vi "HFRR ADV v09.vi"() -> ()   [LabVIEW 2025] (continued)
                    n2657 = Get Date/Time In Seconds() -> (seconds since 1Jan1904=w3395:timestamp)
                    n2658 = To Double Precision Float(number=w3395) -> (double precision float=w3393:dbl)
                    n2659 = local write "acq timer"(w3393) -> ()
                    n2660 = local write "act save time"(w3393) -> ()
                  }
                }
                n2661 = call "Elapsed Time"("Time Target (s)"="Countdown", "Reset"=w3299) -> ("Elapsed Time (s)"=w3304:dbl, "Time has Elapsed"=w3302:bool)  [unwired: 10 in, 6 out]
                "Countdown 2" <- w3304
                n2662 = Subtract(x=w3304, y=2.0) -> (x-y=w3307:dbl)
                n2663 = Less?(x=w3307, y="Countdown") -> (x < y?=w3305:bool)
                n2664 = And(x=w3305, y=w3302) -> (x .and. y?=w3301:bool)
                n2665 = case shown="True" w3301 {
                  frame False {
                  }
                  frame True {
                    (unwired) dbl[] [] ("History Data")
                    n2666 = local write "Engage"(FALSE ("Engage")) -> ()
                    n2667 = local write "RUN"(TRUE ("RUN")) -> ()
                    n2668 = local read "Humidity ( %RH )"() -> (→"Rh Before":dbl)
                  }
                }
                n2669 = local read "Test \nStatus"() -> (w3297:bool)
                n2670 = Select(t=w3295, s=w3297, f=0.0) -> (s? t:f=w3296:dbl)
                n2671 = local write "Frequency ( Hz )"(w3296) -> ()
                n2672 = local write "Freq"(w3296) -> ()
              }
              frame #1 {
                w3418 = 1000000.0 ("x")
                # "Elapsed time\ncof\nstroke\nAir temp\nTemp\nHumidity"
                # "acq timer\n\nact save time"
                # "convert to microseconds"
                n2673 = local read "COUNT"() -> (w3401:i32)
                n2674 = local read "Rate"() -> (w3414:dbl)
                n2675 = Divide(x=w3418, y=w3414) -> (x/y=w3419:dbl)
                n2676 = Greater Or Equal?(x=w3401, y=250) -> (x >= y?=w3400:bool)
                n2677 = Get Date/Time In Seconds() -> (seconds since 1Jan1904=w3421:timestamp)
                n2678 = case shown="True" w3400 {
                  frame False {
                    n2679 = local read "COUNT"() -> (w3422:i32)
                    n2680 = Increment(x=w3422) -> (x+1=w3423:i32)
                    n2681 = local write "COUNT"(w3423) -> ()
                  }
                  frame True {
                    n2682 = local write "COUNT"(0 ("COUNT")) -> ()
                  }
                }
                n2683 = local read "Samplingtime 2"() -> (w3399:dbl)
                n2684 = local read "act save time"() -> (w3416:dbl)
                n2685 = Divide(x=w3419, y=w3418) -> (x/y=w3417:dbl)
                n2686 = To Double Precision Float(number=w3421) -> (double precision float=w3410:dbl)
                n2687 = Add(x=w3416, y=w3399) -> (x+y=w3415:dbl)
                n2688 = local read "acq timer"() -> (w3420:dbl)
                n2689 = local read "COUNT"() -> (w3403:i32)
                n2690 = Greater Or Equal?(x=w3410, y=w3415) -> (x >= y?=w3398:bool)
                n2691 = Multiply(x=w3417, y=w3403) -> (x*y=w3409:dbl)
                n2692 = Subtract(x=w3410, y=w3420) -> (x-y=w3412:dbl)
                n2693 = local read "Save"() -> (w3413:bool)
                n2694 = Add(x=w3412, y=w3409) -> (x+y=w3396:dbl)
                "Elapsed time 3" <- w3396
                n2695 = And(x=w3398, y=w3413) -> (x .and. y?=w3411:bool)
                n2696 = Divide(x=w3396, y=60.0) -> (x/y=w3407:dbl)
                n2697 = local read "Test \nStatus"() -> (w3397:bool)
                n2698 = local read "clk"() -> (w3404:dbl)
                n2699 = Equal?(x=w3404, y=10.0) -> (x = y?=w3406:bool)
                n2700 = case shown="True" w3411 {
                  tunnel: w3410 -> [_ w3525]
                  tunnel: [FALSE ("Boolean 2") TRUE ("Boolean 2")] -> _
                  frame False {
                  }
                  frame True {
                    w3472 = ";" ("Substring")
                    # "Pid out/\nFreq response value"
                    n2701 = local write "act save time"(w3525) -> ()
                    n2702 = local read "FILE"() -> (w3466:string)
                    n2703 = call "file check.vi"("file name in"=w3466) -> ("error out"=w3469:errorcluster, "file name out"=w3464:string)  [unwired: 9 in]
                    n2704 = call "FILE PATH CREATION.vi"("error in"=w3469, "FILE NAME :"=w3464) -> ("FILE OUT"=w3467:path)  [unwired: 8 in, 1 out]
                    n2705 = Concatenate Strings(w3464, ".dgf" ("Substring")) -> (w3468:string)
                    n2706 = local read "Set Strk"() -> (w3496:dbl)
                    n2707 = local read "Stroke"() -> (w3487:dbl)
                    n2708 = local read "FF 2"() -> (→"Frictional Force ( N )" →"Frictional Force ( N )":dbl)
                    n2709 = Build Path(base path=w3467, name or relative path=w3468) -> (appended path=w3463:path)
                    n2710 = Subtract(x=w3487, y=w3496) -> (x-y=w3493:dbl)
                    n2711 = local read "COF 2"() -> (w3478:dbl)
                    "cof" <- w3478
                    "Coefficient of Friction" <- w3478
                    "COF 4" <- w3478
                    "Coefficient of Friction" <- w3478
                    n2712 = Multiply(x=w3493, y=0.05) -> (x*y=w3495:dbl)
                    n2713 = local read "TEMP"() -> (w3482:dbl)
                    "Temp" <- w3482
                    "Temperature ( Deg C )" <- w3482
                    n2714 = Add(x=w3495, y=w3496) -> (x+y=w3476:dbl)
                    "Stroke Ln" <- w3476
                    "Disp" <- w3476
                    n2715 = local read "ecr"() -> (w3479:dbl)
                    "Electrical Contact Resistance ( % )" <- w3479
                    n2716 = local read "Humidity ( %RH )"() -> (w3481:dbl)
                    "Humidity ( %RH )" <- w3481
                    "Humidity ( %RH )" <- w3481
                    n2717 = local read "Frequency ( Hz )"() -> (w3489:dbl)
                    n2718 = local read "Elapsed time"() -> (w3518:dbl)
                    n2719 = disable-structure shown="Disabled" {
                      frame Disabled {
                        n2720 = local read "ecr 3"() -> ()  [unwired: 1 in]
                      }
                      frame Enabled {
                      }
                    }
                    n2721 = local read "AIR TEMP"() -> (w3486:dbl)
                    n2722 = local read "PID-out"() -> (w3492:dbl)
                    n2723 = local write "Temperature ( Deg C )"(w3482) -> ()
                    n2724 = local write "Electrical Contact Resistance ( % )"(w3479) -> ()
                    n2725 = Number To Fractional String(number=w3476, width (-)=i16 9 ("precision (6)"), precision (6)=i16 6) -> (F-format string=w3511:string)  [unwired: 1 in]
                    n2726 = Number To Fractional String(number=w3486, width (-)=i16 9 ("precision (6)"), precision (6)=i16 3) -> (F-format string=w3510:string)  [unwired: 1 in]
                    n2727 = Number To Fractional String(number=w3482, width (-)=i16 9 ("precision (6)"), precision (6)=i16 3) -> (F-format string=w3507:string)  [unwired: 1 in]
                    n2728 = Number To Fractional String(number=w3481, width (-)=i16 9 ("precision (6)"), precision (6)=i16 3) -> (F-format string=w3504:string)  [unwired: 1 in]
                    n2729 = Number To Fractional String(number=w3479, width (-)=i16 9 ("precision (6)"), precision (6)=i16 3) -> (F-format string=w3501:string)  [unwired: 1 in]
                    n2730 = Number To Fractional String(number=w3492, width (-)=i16 9 ("precision (6)"), precision (6)=i16 3) -> (F-format string=w3497:string)  [unwired: 1 in]
                    n2731 = Number To Fractional String(number=w3489, width (-)=i16 9 ("precision (6)"), precision (6)=i16 3) -> (F-format string=w3488:string)  [unwired: 1 in]
                    n2732 = Number To Fractional String(number=w3478, width (-)=i16 9 ("precision (6)"), precision (6)=i16 6) -> (F-format string=w3519:string)  [unwired: 1 in]
                    n2733 = Number To Fractional String(number=w3518, width (-)=i16 14 ("precision (6)"), precision (6)=i16 3) -> (F-format string=w3520:string)  [unwired: 1 in]
                    n2734 = Bundle("y"=1.02, w3476, "y"=0.98) -> (w3480:cluster{"y":dbl, dbl, "y":dbl})  [unwired: 1 in]
                    n2735 = Number To Fractional String(number="Ambient Humidity :", width (-)=i16 9 ("precision (6)"), precision (6)=i16 6) -> (F-format string=w3470:string)  [unwired: 1 in]
                    n2736 = local read "RUN"() -> (w3477:bool)
                    n2737 = case shown="True" w3477 {
                      tunnel: w3480 -> [_ w3530]
                      tunnel: w3476 -> [_ w3529]
                      tunnel: w3476 -> [_ w3528]
                      tunnel: w3476 -> [_ w3527]
                      frame False {
                      }
                      frame True {
                        "Stroke ( mm )" <- w3530
                        "Stroke ( mm )" <- w3530
                        "Stroke 4" <- w3529
                        "Stroke 3" <- w3528
                        "Stroke 2" <- w3527
                      }
                    }
                    n2738 = Concatenate Strings(w3520, w3472, w3519, w3472, w3511, w3472, w3510, w3472, w3507, w3472, w3504, w3472, w3501, w3472, w3497, w3472, w3488, w3472, w3470, "\r") -> (w3517:string)
                    n2739 = call <vilib>:"Write Characters To File.vi"("append to file? (new file:F)"=TRUE, "character string"=w3517, "file path (dialog if empty)"=w3463) -> ()  [unwired: 2 in, 1 out]
                    "refresh flag" <- TRUE ("refresh flag")
                  }
                }
                n2740 = case shown="True" w3397 {
                  tunnel: w3407 -> [_ w3433]
                  tunnel: w3412 -> [_ w3443]
                  tunnel: [0.0 w3439] -> _
                  tunnel: w3406 -> [_ w3438]
                  tunnel: [0.0 w3437] -> _
                  tunnel: w3396 -> [_ w3437]
                  tunnel: w3410 -> [w3426 _]
                  frame False {
                    n2741 = local write "acq timer"(w3426) -> ()
                    n2742 = local write "Test Duration Status"(0.0 ("Test Duration Status")) -> ()
                  }
                  frame True {
                    n2743 = local read "Set Hz"() -> (w3440:dbl)
                    n2744 = local write "Elapsed time"(w3433) -> ()
                    n2745 = local read "test time"() -> (w3432:dbl)
                    n2746 = Multiply(x=w3443, y=w3440) -> (x*y=w3442:dbl)
                    n2747 = case shown="False" w3438 {
                      tunnel: w3442 -> [w3444 _]
                      tunnel: [w3444 1.0] -> w3439
                      frame False {
                        n2748 = local write "Cycles elapsed"(w3444) -> ()
                      }
                      frame True {
                      }
                    }
                    n2749 = Greater?(x=w3433, y=w3432) -> (0:w3441:bool)
                    n2750 = Subtract(x=w3432, y=w3433) -> (x-y=w3431:dbl)
                    "time" <- w3431
                    n2751 = Multiply(x=w3431, y=60.0) -> (x*y=w3430:dbl)
                    n2752 = local write "Time Remaining"(w3430) -> ()
                    n2753 = local write "Remaining Time"(w3430) -> ()
                    n2754 = case shown="True" w3441 {
                      frame False {
                      }
                      frame True {
                        w3446 = T15."Enabled" ("Disabled")
                        w3450 = "" ("FILE")
                        w3451 = TRUE ("Visible")
                        n2755 = local write "Humidity"(FALSE ("Humidity")) -> ()
                        n2756 = local write "RUN"(FALSE ("OK Button 2")) -> ()
                        n2757 = local write "Heater Button"(FALSE ("Heater Button")) -> ()
                        n2758 = local write "Auto Start Test"(FALSE ("Auto Start Test")) -> ()
                        n2759 = local write "TestCompFlg"(TRUE ("StpFlg")) -> ()
                        n2760 = local read "Humidity ( %RH )"() -> (→"Rh After":dbl)
                        n2761 = property on="STOP 2" class="Bool (strict)"("Disabled"=u8 0) -> ()  [unwired: 2 in, 2 out]
                        n2762 = local read "EVENT LOG"() -> (w3456:string)
                        n2763 = call "Event Log.vi"("Content"="Test Completed", "EVENT LOG"=w3456) -> ("EVENT LOG"=w3455:string)  [unwired: 8 in, 1 out]
                        n2764 = property on="RUN" class="Bool (strict)"("Visible"=w3451) -> ()  [unwired: 2 in, 2 out]
                        n2765 = property on="Auto Start Test" class="Bool (strict)"("Visible"=w3451) -> ()  [unwired: 2 in, 2 out]
                        n2766 = local write "Batch Ref Num :"(w3450) -> ()
                        n2767 = local write "FILE"(w3450) -> ()
                        n2768 = local write "EVENT LOG"(w3455) -> ()
                        n2769 = local write "TEST FILE NAM,E SAVED"(FALSE ("TEST FILE NAM,E SAVED")) -> ()
                        n2770 = local write "Fuel Discription :"(w3450) -> ()
                        n2771 = local write "Remarks :"(w3450) -> ()
                        n2772 = local write "Main Dashboard Buttons"(T1."Imaging" ("Main Dashboard Buttons")) -> ()
                        n2773 = local write "Main Tab"(T2."Adv Scar" ("Main Tab")) -> ()
                        n2774 = property on="FRICVALZ 2" class="Bool (strict)"("DisabledEnum"=w3446) -> ()  [unwired: 2 in, 2 out]
                        n2775 = property on="FRICVALZ 3" class="Bool (strict)"("DisabledEnum"=w3446) -> ()  [unwired: 2 in, 2 out]
                        n2776 = property on="FRICVALZ 4" class="Bool (strict)"("DisabledEnum"=w3446) -> ()  [unwired: 2 in, 2 out]
                      }
                    }
                    n2777 = Divide(x=w3433, y=w3432) -> (x/y=w3436:dbl)
                    n2778 = Multiply(x=w3436, y=100.0) -> (x*y=w3434:dbl)
                    n2779 = local write "Test Duration Status"(w3434) -> ()
                  }
                }
              }
              frame #2 {
                n2780 = case shown="True" "Heater Button" {
                  tunnel: [0.0 ("output") w3554] -> w3531
                  frame False {
                    w3534 = TRUE ("tmpchk")
                    n2781 = local read "TEMP"() -> (w3535:dbl)
                    n2782 = local write "Temp ini"(w3535) -> ()
                    n2783 = local write "Reset 4"(w3534) -> ()
                    n2784 = local write "tmpchk"(w3534) -> ()
                    n2785 = local write "reinit"(TRUE ("reinit")) -> ()
                    n2786 = local write "manual temp log"(TRUE ("manual temp log")) -> ()
                  }
                  frame True {
                    # "Logic to turn off\nthe heater when \ntemp is not rising.\nTime - 60 sec\nDelta t- 5°c"
                    n2787 = local read "Temp ini"() -> (w3542:dbl)
                    n2788 = local read "Auto Start Test"() -> (w3538:bool)
                    n2789 = Less?(x=w3542, y=53.0) -> (x < y?=w3540:bool)
                    n2790 = case shown="False" w3538 {
                      frame False {
                        n2791 = local read "Set Temp"() -> (w3565:dbl)
                        n2792 = local read "TEMP"() -> (w3564:dbl)
                        n2793 = Subtract(x=w3565, y=w3564) -> (x-y=w3563:dbl)
                        n2794 = Absolute Value(x=w3563) -> (abs(x)=w3562:dbl)
                        n2795 = Less?(x=w3562, y=0.5) -> (x < y?=w3560:bool)
                        n2796 = case shown="True" w3560 {
                          tunnel: "manual temp log" -> [_ w3566]
                          frame False {
                          }
                          frame True {
                            n2797 = case shown="True" w3566 {
                              selector: w3566 -> [_ w3567]
                              frame False {
                              }
                              frame True {
                                # "#Event log"
                                n2798 = Not(x=w3567) -> (.not. x?=w3568:bool)
                                n2799 = local write "manual temp log"(w3568) -> ()
                                n2800 = local read "EVENT LOG"() -> (w3571:string)
                                n2801 = call "Event Log.vi"("Content"="Target Temperature reached", "EVENT LOG"=w3571) -> ("EVENT LOG"=w3570:string)  [unwired: 8 in, 1 out]
                                n2802 = local write "EVENT LOG"(w3570) -> ()
                              }
                            }
                          }
                        }
                      }
                      frame True {
                        n2803 = local write "manual temp log"(TRUE ("manual temp log")) -> ()
                      }
                    }
                    n2804 = And(x="tmpchk", y=w3540) -> (x .and. y?=w3543:bool)
                    n2805 = case shown="True" w3543 {
                      frame False {
                      }
                      frame True {
                        n2806 = call "Elapsed Time8"("Time Target (s)"=300.0, "Reset"="Reset 4") -> ("Time has Elapsed"=w3573:bool)  [unwired: 10 in, 7 out]
                        n2807 = flat-sequence {
                          tunnel: w3573 -> [_]
                          frame #0 {
                            n2808 = local write "Reset 4"(FALSE ("Reset 4")) -> ()
                          }
                        }
                        n2809 = case shown="True" w3573 {
                          frame False {
                          }
                          frame True {
                            n2810 = local read "Temp ini"() -> (w3580:dbl)
                            n2811 = Add(x=w3580, y=5.0) -> (x+y=w3578:dbl)
                            n2812 = local read "TEMP"() -> (w3581:dbl)
                            n2813 = Greater?(x=w3581, y=w3578) -> (0:w3579:bool)
                            n2814 = case shown="False" w3579 {
                              frame False {
                                n2815 = local write "Heater Button"(FALSE ("Heater Button")) -> ()
                              }
                              frame True {
                                n2816 = local write "tmpchk"(FALSE ("tmpchk")) -> ()
                              }
                            }
                          }
                        }
                      }
                    }
                    n2817 = local read "Set Temp"() -> (w3551:dbl)
                    n2818 = local read "TEMP"() -> (w3545:dbl)
                    n2819 = call-poly <vilib>:"PID.vi"("reinitialize? (F)"="reinit", "output range"="output range", "dt (s)"=-1.0, "PID gains"="Temp PID gains", "process variable"=w3545, "setpoint"=w3551) -> ("output"=w3548:dbl)  [unwired: 4 in, 1 out]
                    n2820 = Subtract(x=w3551, y=w3545) -> (x-y=w3553:dbl)
                    n2821 = Add(x=w3551, y=0.5) -> (x+y=w3549:dbl)
                    n2822 = Greater Or Equal?(x=w3545, y=w3549) -> ()  [unwired: 1 out]
                    n2823 = Select(t=0.0, s=FALSE, f=w3548) -> (s? t:f=w3547:dbl)
                    "PID output" <- w3547
                    n2824 = flat-sequence {
                      tunnel: w3547 -> [w3584]
                      tunnel: [w3584] -> w3554
                      frame #0 {
                        n2825 = local write "reinit"(FALSE ("reinit")) -> ()
                      }
                    }
                    n2826 = Bundle(w3553, "output"=w3547, "TEMP"=w3545) -> (→"gTEMP 3":cluster{dbl, "output":dbl, "TEMP":dbl})  [unwired: 1 in]
                  }
                }
                "PID-out" <- w3531
              }
              frame #3 {
                n2827 = local read "TEMP"() -> (w3586:dbl)
                n2828 = Greater Or Equal?(x=w3586, y="Set Temp 2") -> (x >= y?=w3591:bool)
                n2829 = case shown="True" w3591 {
                  tunnel: [FALSE TRUE] -> w3589
                  frame False {
                  }
                  frame True {
                  }
                }
                "Status 13" <- w3589
                n2830 = And(x=w3589, y="trip1 8") -> (x .and. y?=w3588:bool)
                n2831 = case shown="True" w3588 {
                  frame False {
                    n2832 = local write "Heater Trip Temp"(TRUE ("Heater Trip Temp")) -> ()
                  }
                  frame True {
                    w3594 = FALSE ("OK Button 2")
                    n2833 = case shown="True" "Heater Trip Temp" {
                      selector: "Heater Trip Temp" -> [_ w3596]
                      frame False {
                      }
                      frame True {
                        n2834 = Not(x=w3596) -> (.not. x?=w3595:bool)
                        n2835 = local read "EVENT LOG"() -> (w3599:string)
                        n2836 = local write "Heater Trip Temp"(w3595) -> ()
                        n2837 = call "Event Log.vi"("Content"="Heater Trip", "EVENT LOG"=w3599) -> ("EVENT LOG"=w3598:string)  [unwired: 8 in, 1 out]
                        n2838 = local write "EVENT LOG"(w3598) -> ()
                      }
                    }
                    n2839 = local write "RUN"(w3594) -> ()
                    n2840 = property on="Auto Start Test" class="Bool (strict)"("Value"=w3594) -> ()  [unwired: 2 in, 2 out]
                    n2841 = local write "Heater Button"(w3594) -> ()
                  }
                }
              }
            }
            n2842 = case shown="False" w3290 {
              frame False {
                n2843 = disable-structure shown="Enabled" {
                  frame Enabled {
                    n2844 = stacked-sequence {
                      frame #0 {
                        n2845 = local write "RUN"(FALSE ("OK Button 2")) -> ()
                      }
                      frame #1 {
                      }
                    }
                  }
                  frame Disabled {
                  }
                }
              }
              frame True {
              }
            }
          }
        }
        n2846 = local read "airtempflg"() -> (w3082:bool)
        n2847 = Or(x=w3082, y=w3080) -> (x .or. y?=w3083:bool)
        n2848 = Insert Into Array(array=string[] ["Air Temperature has reached set value,", "Humidity has reached set value,", "Sample Temperaturehas reached set value,", ""], index=0, new element="") -> (w3068:string[])
        n2849 = Build Array(w3073, w3072, w3071) -> (w3069:i32[])
        n2850 = disable-structure shown="Disabled" {
          disable-tunnel: w3083 -> [w3160 _]
          disable-tunnel: w3078 -> [w3159 _]
          disable-tunnel: w3076 -> [w3158 _]
          frame Disabled {
            n2851 = Compound Arithmetic op=AND(w3160, w3159, w3158) -> ()  [unwired: 1 out]
            n2852 = case shown="True" {
              selector: _ -> [_ _]
              frame False {
              }
              frame True {
                w3161 = FALSE ("autostrtflg")
                n2853 = local write "RUN"(TRUE ("RUN")) -> ()
                n2854 = local write "autostrtflg"(w3161) -> ()
                n2855 = local write "autostart"(w3161) -> ()
                n2856 = local write "String 14"(" Running....." ("String 14")) -> ()
              }
            }
          }
          frame Enabled {
          }
        }
        n2857 = for {
          tunnel: w3069 -> [w3211] mode=indexing
          tunnel: w3068 -> [w3210]
          shift-right: [w3207] -> w3067
          shift-left: "" -> [w3209]
          n2858 = Index Array(array=w3210, index=w3211) -> (element=w3208:string)
          n2859 = Concatenate Strings(w3208, w3209) -> (w3207:string)
        }
        n2860 = local write "autostart 2"(w3067) -> ()
        n2861 = local read "Reset Graph"() -> (w3056:bool)
        n2862 = case shown="True" w3056 {
          selector: w3056 -> [_ w3110]
          frame False {
          }
          frame True {
            w3124 = 0.0 ("X Scale.Range:Maximum")
            n2863 = Not(x=w3110) -> (.not. x?=w3109:bool)
            n2864 = local write "Reset Graph"(w3109) -> ()
            n2865 = property on="Electrical Contact Resistance ( % )" class="WFChart (strict)"("XScale.Maximum"=600.0 ("X Scale.Range:Maximum"), "XScale.Minimum"=0.0 ("X Scale.Range:Minimum"), "YScale.Maximum"=100.0 ("Y Scale.Range:Maximum"), "YScale.Minimum"=0.0 ("Y Scale.Range:Minimum")) -> ()  [unwired: 2 in, 2 out]
            n2866 = property on="Frictional Force ( N )" class="WFChart (strict)"("XScale.Maximum"=600.0 ("X Scale.Range:Maximum"), "XScale.Minimum"=0.0 ("X Scale.Range:Minimum"), "YScale.Maximum"=100.0 ("Y Scale.Range:Maximum"), "YScale.Minimum"=0.0 ("Y Scale.Range:Minimum")) -> ()  [unwired: 2 in, 2 out]
            n2867 = property on="Temperature ( Deg C )" class="WFChart (strict)"("XScale.Maximum"=600.0 ("X Scale.Range:Maximum"), "XScale.Minimum"=0.0 ("X Scale.Range:Minimum"), "YScale.Maximum"=100.0 ("Y Scale.Range:Maximum"), "YScale.Minimum"=0.0 ("Y Scale.Range:Minimum")) -> ()  [unwired: 2 in, 2 out]
            n2868 = property on="Humidity ( %RH )" class="WFChart (strict)"("XScale.Maximum"=600.0 ("X Scale.Range:Maximum"), "XScale.Minimum"=0.0 ("X Scale.Range:Minimum"), "YScale.Maximum"=100.0 ("Y Scale.Range:Maximum"), "YScale.Minimum"=0.0 ("Y Scale.Range:Minimum")) -> ()  [unwired: 2 in, 2 out]
            n2869 = property on="Stroke ( mm )" class="WFChart (strict)"("XScale.Maximum"=600.0 ("X Scale.Range:Maximum"), "XScale.Minimum"=0.0 ("X Scale.Range:Minimum"), "YScale.Maximum"=100.0 ("Y Scale.Range:Maximum"), "YScale.Minimum"=0.0 ("Y Scale.Range:Minimum")) -> ()  [unwired: 2 in, 2 out]
            n2870 = property on="Coefficient of Friction" class="WFChart (strict)"("XScale.Maximum"=600.0 ("X Scale.Range:Maximum"), "XScale.Minimum"=0.0 ("X Scale.Range:Minimum"), "YScale.Maximum"=100.0 ("Y Scale.Range:Maximum"), "YScale.Minimum"=0.0 ("Y Scale.Range:Minimum")) -> ()  [unwired: 2 in, 2 out]
            n2871 = property on="Electrical Contact Resistance ( % )" class="WFChart (strict)"("XScale.Minimum"=0.0 ("X Scale.Range:Minimum"), "XScale.Maximum"=600.0 ("X Scale.Range:Maximum"), "YScale.Minimum"=0.0 ("Y Scale.Range:Minimum"), "YScale.Maximum"=100.0 ("Y Scale.Range:Maximum")) -> ()  [unwired: 2 in, 2 out]
            n2872 = property on="Temperature ( Deg C )" class="WFChart (strict)"("XScale.Minimum"=0.0 ("X Scale.Range:Minimum"), "XScale.Maximum"=600.0 ("X Scale.Range:Maximum"), "YScale.Minimum"=0.0 ("Y Scale.Range:Minimum"), "YScale.Maximum"=100.0 ("Y Scale.Range:Maximum")) -> ()  [unwired: 2 in, 2 out]
            n2873 = property on="Coefficient of Friction" class="WFChart (strict)"("XScale.Minimum"=0.0 ("X Scale.Range:Minimum"), "XScale.Maximum"=600.0 ("X Scale.Range:Maximum"), "YScale.Maximum"=1.0 ("X Scale.Range:Minimum"), "YScale.Minimum"=0.0 ("X Scale.Range:Minimum")) -> ()  [unwired: 2 in, 2 out]
            n2874 = property on="Frictional Force ( N )" class="WFChart (strict)"("XScale.Maximum"=600.0 ("X Scale.Range:Maximum"), "XScale.Minimum"=w3124, "YScale.Maximum"=10.0 ("Y Scale.Range:Maximum"), "YScale.Minimum"=w3124) -> ()  [unwired: 2 in, 2 out]
            n2875 = property on="Stroke ( mm )" class="WFChart (strict)"("XScale.Maximum"=600.0 ("X Scale.Range:Maximum"), "XScale.Minimum"=0.0 ("X Scale.Range:Minimum"), "YScale.Maximum"=100.0 ("Y Scale.Range:Maximum"), "YScale.Minimum"=0.0 ("Y Scale.Range:Minimum")) -> ()  [unwired: 2 in, 2 out]
            n2876 = property on="Humidity ( %RH )" class="WFChart (strict)"("XScale.Maximum"=600.0 ("X Scale.Range:Maximum"), "XScale.Minimum"=0.0 ("X Scale.Range:Minimum"), "YScale.Maximum"=100.0 ("Y Scale.Range:Maximum"), "YScale.Minimum"=0.0 ("Y Scale.Range:Minimum")) -> ()  [unwired: 2 in, 2 out]
          }
        }
      }
      frame "Compare Files" {
        # "Elapsed time\ncof\nstroke\nAir temp\nTemp\nHumidity"
        n2877 = case shown="True" "RSTV1 2" {
          frame False {
          }
          frame True {
            n2878 = property on="Humidity ( %RH )" class="XYGraph (strict)"("Y Scale.Display Format:Precision"=u8 0 ("Y Scale.Format & Precision:Precision")) -> ()  [unwired: 2 in, 2 out]
            n2879 = property on="Humidity ( %RH )" class="XYGraph (strict)"("X Scale.Range:Minimum"=0.0, "X Scale.Range:Maximum"=75.0, "Y Scale.Range:Minimum"=48.0, "Y Scale.Range:Maximum"=58.0) -> ()  [unwired: 2 in, 2 out]
          }
        }
        n2880 = case shown="True" "RST CP 2" {
          frame False {
          }
          frame True {
            n2881 = property on="XY Graph 13" class="XYGraph (strict)"("Y Scale.Display Format:Precision"=u8 0 ("Y Scale.Format & Precision:Precision")) -> ()  [unwired: 2 in, 2 out]
            n2882 = property on="XY Graph 13" class="XYGraph (strict)"("X Scale.Range:Minimum"=0.0, "X Scale.Range:Maximum"=75.0, "Y Scale.Range:Minimum"=0.0, "Y Scale.Range:Maximum"=100.0) -> ()  [unwired: 2 in, 2 out]
          }
        }
        n2883 = case shown="True" "RST CP" {
          frame False {
          }
          frame True {
            n2884 = property on="Sample Temperature ( °C )" class="XYGraph (strict)"("Y Scale.Display Format:Precision"=u8 2 ("Y Scale.Format & Precision:Precision")) -> ()  [unwired: 2 in, 2 out]
            n2885 = property on="Sample Temperature ( °C )" class="XYGraph (strict)"("X Scale.Range:Minimum"=0.0, "X Scale.Range:Maximum"=75.0, "Y Scale.Range:Minimum"=58.0, "Y Scale.Range:Maximum"=62.0) -> ()  [unwired: 2 in, 2 out]
          }
        }
        n2886 = case shown="True" "RSTV1 3" {
          frame False {
          }
          frame True {
            n2887 = property on="Air Temperature  ( °C )" class="XYGraph (strict)"("Y Scale.Display Format:Precision"=u8 2 ("Y Scale.Format & Precision:Precision")) -> ()  [unwired: 2 in, 2 out]
            n2888 = property on="Air Temperature  ( °C )" class="XYGraph (strict)"("X Scale.Range:Minimum"=0.0 ("Y Scale.Range:Minimum"), "X Scale.Range:Maximum"=75.0 ("Y Scale.Range:Maximum"), "Y Scale.Range:Minimum"=20.0 ("X Scale.Range:Minimum"), "Y Scale.Range:Maximum"=26.0 ("X Scale.Range:Maximum")) -> ()  [unwired: 2 in, 2 out]
          }
        }
        n2889 = case shown="True" "RSTV1 4" {
          frame False {
          }
          frame True {
            n2890 = property on="Stroke ( mm )" class="XYGraph (strict)"("Y Scale.Display Format:Precision"=u8 2 ("Y Scale.Format & Precision:Precision")) -> ()  [unwired: 2 in, 2 out]
            n2891 = property on="Stroke ( mm )" class="XYGraph (strict)"("X Scale.Range:Minimum"=0.0 ("Y Scale.Range:Maximum"), "X Scale.Range:Maximum"=75.0 ("X Scale.Range:Minimum"), "Y Scale.Range:Minimum"=0.98, "Y Scale.Range:Maximum"=1.02) -> ()  [unwired: 2 in, 2 out]
          }
        }
        n2892 = case shown="True" "rstv2" {
          frame False {
          }
          frame True {
            n2893 = property on="Coefficient Of Friction" class="XYGraph (strict)"("Y Scale.Display Format:Precision"=u8 3 ("Y Scale.Format & Precision:Precision")) -> ()  [unwired: 2 in, 2 out]
            n2894 = property on="Coefficient Of Friction" class="XYGraph (strict)"("X Scale.Range:Minimum"=0.0 ("Y Scale.Range:Maximum"), "X Scale.Range:Maximum"=75.0, "Y Scale.Range:Minimum"=0.0, "Y Scale.Range:Maximum"=1.0 ("X Scale.Range:Minimum")) -> ()  [unwired: 2 in, 2 out]
          }
        }
        n2895 = case shown="True" "RST CP 3" {
          frame False {
          }
          frame True {
            n2896 = property on="Air Temp ( °C ) vs Humidity ( % RH )" class="XYGraph (strict)"("X Scale.Range:Minimum"=18.0, "X Scale.Range:Maximum"=28.0 ("X Scale.Range:Minimum"), "Y Scale.Range:Minimum"=30.0 ("X Scale.Range:Minimum"), "Y Scale.Range:Maximum"=70.0 ("X Scale.Range:Minimum")) -> ()  [unwired: 2 in, 2 out]
          }
        }
        n2897 = case shown="True" "OPEN 1" {
          frame False {
          }
          frame True {
            (unwired) 0  # existing file
            w3874 = "Choose a datalog file to open"  # prompt
            n2898 = local write "OPEN 1"(FALSE ("OPEN 1")) -> ()
            n2899 = String To Path(string="C:\\LAB-IQ\\Data\\") -> (path=w3859:path)
            n2900 = File Dialog(6:"*.dgf" ("pattern"), 7:w3874, 11:w3859) -> (0:w3857:errorcluster, 3:w3865:path)  [unwired: 4 in, 2 out]
            n2901 = Unbundle(w3857) -> ()  [unwired: 3 out]
            n2902 = Strip Path(path=w3865) -> (name=w3864:string)  [unwired: 1 out]
            n2903 = Path To String(path=w3865) -> (string=w3860:string)
            "string1" <- w3860
            n2904 = Match Pattern(string=w3864, regular expression=".dgf") -> (before substring=→"String Control":string)  [unwired: 1 in, 3 out]
            n2905 = Match Pattern(string=w3860, regular expression=".dgf" ("substring (\"\")")) -> (before substring=w3870:string)  [unwired: 1 in, 3 out]
            n2906 = Concatenate Strings(w3870, ".duf" ("Substring")) -> (w3866:string)
            n2907 = String To Path(string=w3866) -> (path=w3871:path)
            n2908 = call <vilib>:"Read Characters From File.vi"("file path (dialog if empty)"=w3871, "start of read offset (chars.:0)"=60 ("start of read offset (chars.: 0)")) -> ("character string"=→"String Control 2":string)  [unwired: 4 in, 3 out]
          }
        }
        n2909 = case shown="True" "OPEN 2" {
          frame False {
          }
          frame True {
            (unwired) 0  # existing file
            w3892 = "Choose a datalog file to open"  # prompt
            n2910 = local write "OPEN 2"(FALSE ("OPEN 1")) -> ()
            n2911 = String To Path(string="C:\\LAB-IQ\\Data\\") -> (path=w3877:path)
            n2912 = File Dialog(6:"*.dgf" ("pattern"), 7:w3892, 11:w3877) -> (0:w3875:errorcluster, 3:w3883:path)  [unwired: 4 in, 2 out]
            n2913 = Unbundle(w3875) -> ()  [unwired: 3 out]
            n2914 = Strip Path(path=w3883) -> (name=w3881:string)  [unwired: 1 out]
            n2915 = Path To String(path=w3883) -> (string=w3878:string)
            "string1 2" <- w3878
            n2916 = Match Pattern(string=w3881, regular expression=".dgf") -> (before substring=→"String Control 3":string)  [unwired: 1 in, 3 out]
            n2917 = Match Pattern(string=w3878, regular expression=".dgf" ("substring (\"\")")) -> (before substring=w3889:string)  [unwired: 1 in, 3 out]
            n2918 = Concatenate Strings(w3889, ".duf" ("Substring")) -> (w3886:string)
            n2919 = String To Path(string=w3886) -> (path=w3884:path)
            n2920 = call <vilib>:"Read Characters From File.vi"("file path (dialog if empty)"=w3884, "start of read offset (chars.:0)"=60 ("start of read offset (chars.: 0)")) -> ("character string"=→"String Control 4":string)  [unwired: 4 in, 3 out]
          }
        }
        n2921 = case shown="True" "OPEN 3" {
          frame False {
          }
          frame True {
            (unwired) 0  # existing file
            w3910 = "Choose a datalog file to open"  # prompt
            n2922 = local write "OPEN 3"(FALSE ("OPEN 1")) -> ()
            n2923 = String To Path(string="C:\\LAB-IQ\\Data\\") -> (path=w3895:path)
            n2924 = File Dialog(6:"*.dgf" ("pattern"), 7:w3910, 11:w3895) -> (0:w3893:errorcluster, 3:w3901:path)  [unwired: 4 in, 2 out]
            n2925 = Unbundle(w3893) -> ()  [unwired: 3 out]
            n2926 = Strip Path(path=w3901) -> (name=w3899:string)  [unwired: 1 out]
            n2927 = Path To String(path=w3901) -> (string=w3896:string)
            "string1 3" <- w3896
            n2928 = Match Pattern(string=w3899, regular expression=".dgf") -> (before substring=→"String Control 5":string)  [unwired: 1 in, 3 out]
            n2929 = Match Pattern(string=w3896, regular expression=".dgf" ("substring (\"\")")) -> (before substring=w3906:string)  [unwired: 1 in, 3 out]
            n2930 = Concatenate Strings(w3906, ".duf" ("Substring")) -> (w3903:string)
            n2931 = String To Path(string=w3903) -> (path=w3907:path)
            n2932 = call <vilib>:"Read Characters From File.vi"("file path (dialog if empty)"=w3907, "start of read offset (chars.:0)"=60 ("start of read offset (chars.: 0)")) -> ("character string"=→"String Control 6":string)  [unwired: 4 in, 3 out]
          }
        }
        n2933 = case shown="True" "OPEN 4" {
          frame False {
          }
          frame True {
            (unwired) 0  # existing file
            w3928 = "Choose a datalog file to open"  # prompt
            n2934 = local write "OPEN 4"(FALSE ("OPEN 1")) -> ()
            n2935 = String To Path(string="C:\\LAB-IQ\\Data\\") -> (path=w3913:path)
            n2936 = File Dialog(6:"*.dgf" ("pattern"), 7:w3928, 11:w3913) -> (0:w3911:errorcluster, 3:w3919:path)  [unwired: 4 in, 2 out]
            n2937 = Unbundle(w3911) -> ()  [unwired: 3 out]
            n2938 = Strip Path(path=w3919) -> (name=w3917:string)  [unwired: 1 out]
            n2939 = Path To String(path=w3919) -> (string=w3914:string)
            "string1 4" <- w3914
            n2940 = Match Pattern(string=w3917, regular expression=".dgf") -> (before substring=→"String Control 7":string)  [unwired: 1 in, 3 out]
            n2941 = Match Pattern(string=w3914, regular expression=".dgf" ("substring (\"\")")) -> (before substring=w3924:string)  [unwired: 1 in, 3 out]
            n2942 = Concatenate Strings(w3924, ".duf" ("Substring")) -> (w3921:string)
            n2943 = String To Path(string=w3921) -> (path=w3925:path)
            n2944 = call <vilib>:"Read Characters From File.vi"("file path (dialog if empty)"=w3925, "start of read offset (chars.:0)"=60 ("start of read offset (chars.: 0)")) -> ("character string"=→"String Control 8":string)  [unwired: 4 in, 3 out]
          }
        }
      }
      frame "About" {
        # "Elapsed time\ncof\nstroke\nmean pos\nTemp\nHumidity"
        n2945 = disable-structure shown="Disabled" {
          frame Disabled {
            n2946 = case shown="True" "Export" {
              frame False {
              }
              frame True {
                w3950 = "                                      " ("string")
                w3952 = "\r"
                (unwired) i16 6 ("width (-)")
                w4029 = "\r"
                w3961 = "\r"
                n2947 = local write "Export"(FALSE ("Export")) -> ()
                n2948 = local read "String 29"() -> (w3998:string)
                n2949 = local read "String 34"() -> (w3986:string)
                n2950 = local read "String 35"() -> (w3981:string)
                n2951 = local read "String 37"() -> (w3977:string)
                n2952 = local read "String 36"() -> (w3974:string)
                n2953 = local read "String 38"() -> (w3971:string)
                n2954 = local read "String 39"() -> (w3968:string)
                n2955 = Match Pattern(string=w3998, regular expression=".dwm") -> (before substring=w3994:string)  [unwired: 1 in, 3 out]
                "before substring" <- w3994
                n2956 = local read "S 38"() -> (w3989:string)
                n2957 = local read "S 39"() -> (w3982:string)
                n2958 = local read "Temperature before test 2"() -> (w4018:dbl)
                n2959 = local read "Temperature after test 2"() -> (w4023:dbl)
                n2960 = local read "Humidity before test 2"() -> (w4004:dbl)
                n2961 = local read "Humidity after test 2"() -> (w4019:dbl)
                n2962 = local read "MWSD 2"() -> (w4015:dbl)
                n2963 = local read "WS1.4 2"() -> (w4031:dbl)
                n2964 = local read "HCF 2"() -> (w4027:dbl)
                n2965 = local read "AVP 2"() -> (w4016:dbl)
                n2966 = Concatenate Strings("1," ("string"), w3989) -> (w3988:string)
                n2967 = Concatenate Strings("2," ("string"), w3986) -> (w3985:string)
                n2968 = Concatenate Strings("3," ("string"), w3982) -> (w3984:string)
                n2969 = Concatenate Strings("4," ("string"), w3981) -> (w3980:string)
                n2970 = Concatenate Strings("5," ("string"), w3977) -> (w3978:string)
                n2971 = Concatenate Strings("6," ("string"), w3974) -> (w3975:string)
                n2972 = Concatenate Strings("7," ("string"), w3971) -> (w3972:string)
                n2973 = Concatenate Strings("8," ("string"), w3968) -> (w3969:string)
                n2974 = local read "Sample ID"() -> (w4036:string)
                n2975 = case shown="\"xlx\"" "Select File Type" {
                  tunnel: w3994 -> [w4039 w4041 w4043]
                  tunnel: [w4037 w4042 w4044] -> w3993
                  frame "xlx" {
                    n2976 = Concatenate Strings(w4039, ".xls" ("string")) -> (w4037:string)
                  }
                  frame "csv" {
                    n2977 = Concatenate Strings(w4041, ".csv" ("string")) -> (w4042:string)
                  }
                  frame "txt" {
                    n2978 = Concatenate Strings(w4043, ".txt" ("string")) -> (w4044:string)
                  }
                }
                n2979 = local read "Test Date"() -> (w4035:string)
                n2980 = local read "String 45"() -> (w3949:string)
                n2981 = local read "String 31"() -> (w4034:string)
                n2982 = local read "String 32"() -> (w4033:string)
                n2983 = local read "TITTLE"() -> (w3957:string)
                n2984 = Number To Fractional String(number=w4004, width (-)=i16 6, precision (6)=i16 2) -> (F-format string=w4003:string)  [unwired: 1 in]
                n2985 = Number To Fractional String(number=w4018, width (-)=i16 6, precision (6)=i16 2) -> (F-format string=w4024:string)  [unwired: 1 in]
                n2986 = Number To Fractional String(number=w4019, width (-)=i16 6, precision (6)=i16 2) -> (F-format string=w4017:string)  [unwired: 1 in]
                n2987 = Number To Fractional String(number=w4023, width (-)=i16 6, precision (6)=i16 2) -> (F-format string=w4022:string)  [unwired: 1 in]
                n2988 = Number To Fractional String(number=w4015, width (-)=i16 6, precision (6)=i16 2) -> (F-format string=w4013:string)  [unwired: 1 in]
                n2989 = Number To Fractional String(number=w4016, width (-)=i16 6, precision (6)=i16 2) -> (F-format string=w4014:string)  [unwired: 1 in]
                n2990 = Number To Fractional String(number=w4027, width (-)=i16 6, precision (6)=i16 2) -> (F-format string=w4028:string)  [unwired: 1 in]
                n2991 = Number To Fractional String(number=w4031, precision (6)=i16 2) -> (F-format string=w4032:string)  [unwired: 2 in]
                n2992 = local read "s.NO"() -> (w3951:string)
                n2993 = Concatenate Strings("=" ("string"), w3957) -> (w3956:string)
                n2994 = Concatenate Strings("S.No," ("string"), "                                       Parameters" ("string")) -> (w3962:string)
                n2995 = Concatenate Strings(w4029, w3988, w4003, w4029, w3985, w4024, w4029, w3984, w4017, w4029, w3980, w4022, w4029, w3978, w4013, w4029, w3975, w4014, w4029, w3972, w4028, w4029, w3969, w4032) -> (w3991:string)
                n2996 = Concatenate Strings(w3961, "," ("string"), w3949, w3951, w3950, w4033, w4036, w3950, w4034, w4035, w3961) -> (w3959:string)
                n2997 = local read "Tested by"() -> (w3965:string)
                n2998 = local read "String 33"() -> (w3966:string)
                n2999 = Concatenate Strings("," ("string"), "                                                                             " ("string")) -> (w3954:string)
                n3000 = Concatenate Strings(w3956, w3952, w3959, w3952, w3962, w3991, w3952, w3954, w3966, w3965) -> (→"export":string)
                n3001 = String To Path(string=w3993) -> (path=w4000:path)
                n3002 = local read "export"() -> (w3995:string)
                n3003 = call <vilib>:"Write Characters To File.vi"("append to file? (new file:F)"=FALSE, "character string"=w3995, "file path (dialog if empty)"=w4000) -> ()  [unwired: 2 in, 1 out]
              }
            }
          }
          frame Enabled {
          }
        }
        n3004 = case shown="True" "OK Button 17" {
          frame False {
          }
          frame True {
            (unwired) 0  # existing file
            w4253 = "Choose a datalog file to open"  # prompt
            n3005 = local write "OK Button 17"(FALSE ("OK Button 17")) -> ()
            n3006 = local read "String"() -> (w4248:string)
            n3007 = String To Path(string=w4248) -> (path=w4249:path)
            n3008 = File Dialog(6:"*.duf" ("pattern"), 7:w4253, 11:w4249) -> (0:w4240:errorcluster, 3:w4259:path)  [unwired: 4 in, 2 out]
            n3009 = Unbundle(w4240) -> ()  [unwired: 3 out]
            n3010 = Open/Create/Replace File "Open File"(file path (use dialog)=w4259) -> (refnum out=w4251:refnum<file>)  [unwired: 5 in, 2 out]
            n3011 = Strip Path(path=w4259) -> (name=w4257:string)  [unwired: 1 out]
            n3012 = Path To String(path=w4259) -> (string=w4242:string)
            n3013 = while {
              tunnel: w4251 -> [w4263]
              i -> [w4260]
              stop <- w4261 continue-if-true
              (unwired) TRUE ("line mode (F)")
              n3014 = Read from Text File "Read File"(file (use dialog)=w4263) -> (text=w4262:string)  [unwired: 3 in, 3 out]
              n3015 = local write "Numeric 16"(w4260) -> ()
              n3016 = String Length(string=w4262) -> (length=w4265:i32)
              n3017 = Greater?(x=w4265, y=1) -> (0:w4261:bool)
            }
            n3018 = local write "String 29"(w4242) -> ()
            n3019 = Search and Replace String(input string=w4242, search string=".duf", replace string=".dgf" ("replace string (\"\")")) -> (result string=→"String Indicator 4":string)  [unwired: 5 in, 3 out]
            n3020 = Match Pattern(string=w4257, regular expression=".dwm") -> (before substring=w4241:string)  [unwired: 1 in, 3 out]
            "String Indicator" <- w4241
            n3021 = Match Pattern(string=w4242, regular expression=".dwm" ("substring (\"\")")) -> (before substring=w4243:string)  [unwired: 1 in, 3 out]
            "String Indicator 3" <- w4243
            n3022 = local write "TITTLE 2"(w4241) -> ()
            n3023 = String To Path(string=w4243) -> (path=w4250:path)
            "path" <- w4250
            n3024 = call <vilib>:"Read Characters From File.vi"("file path (dialog if empty)"=w4250, "start of read offset (chars.:0)"=60 ("start of read offset (chars.: 0)")) -> ("character string"=→"String Indicator 2":string)  [unwired: 4 in, 3 out]
          }
        }
        n3025 = call <vilib>:"Query Available Printers.vi"() -> ("system configured printers"=w3942:string[])  [unwired: 9 in, 2 out]
        "System Configured Printers 2" <- w3942
        n3026 = local read "OK Button 16"() -> (w3939:bool)
        n3027 = case shown="True" "OK Button 16" {
          frame False {
          }
          frame True {
            n3028 = stacked-sequence {
              frame #0 {
                n3029 = local read "Numeric 16"() -> (w4267:i32)
                n3030 = local write "Numeric 10"(w4267) -> ()
              }
              frame #1 {
                n3031 = local read "S.NO"() -> (→"s.NO":string)
                n3032 = local read "String 29"() -> (w4271:string)
                n3033 = String To Path(string=w4271) -> (path=w4270:path)
                n3034 = Open/Create/Replace File "Open File"(file path (use dialog)=w4270) -> (refnum out=w4272:refnum<file>)  [unwired: 5 in, 2 out]
                n3035 = for {
                  N: 16 -> [_]
                  tunnel: w4272 -> [w4279]
                  i -> [w4275]
                  (unwired) TRUE ("line mode (F)")
                  n3036 = Read from Text File "Read File"(file (use dialog)=w4279) -> (text=w4273:string)  [unwired: 3 in, 3 out]
                  n3037 = Match Pattern(string=w4273, regular expression="(") -> (after substring=w4278:string)  [unwired: 1 in, 3 out]
                  n3038 = Match Pattern(string=w4278, regular expression=")") -> (before substring=w4274:string)  [unwired: 1 in, 3 out]
                  n3039 = case shown="1" w4275 {
                    tunnel: w4274 -> [w4280 w4281 _ _ w4282 w4283 w4284 w4286 w4288 w4290 w4292 w4294 w4296 w4298 _]
                    tunnel: w4273 -> [_ _ _ _ _ _ _ _ _ _ _ _ _ _ _]
                    frame 0 {
                      "TITTLE" <- w4280
                    }
                    frame 1 {
                      "Sample ID" <- w4281
                    }
                    frame 2 {
                    }
                    frame 3 {
                    }
                    frame 4 {
                      "Test Date" <- w4282
                    }
                    frame 5 {
                      "Tested by" <- w4283
                    }
                    frame 6 {
                      n3040 = Fract/Exp String To Number(string=w4284) -> (number=→"Humidity before test 2":dbl)  [unwired: 3 in, 1 out]
                    }
                    frame 7 {
                      n3041 = Fract/Exp String To Number(string=w4286) -> (number=→"Temperature before test 2":dbl)  [unwired: 3 in, 1 out]
                    }
                    frame 8 {
                      n3042 = Fract/Exp String To Number(string=w4288) -> (number=→"Humidity after test 2":dbl)  [unwired: 3 in, 1 out]
                    }
                    frame 9 {
                      n3043 = Fract/Exp String To Number(string=w4290) -> (number=→"Temperature after test 2":dbl)  [unwired: 3 in, 1 out]
                    }
                    frame 10 {
                      n3044 = Fract/Exp String To Number(string=w4292) -> (number=→"MWSD 2":dbl)  [unwired: 3 in, 1 out]
                    }
                    frame 11 {
                      n3045 = Fract/Exp String To Number(string=w4294) -> (number=→"AVP 2":dbl)  [unwired: 3 in, 1 out]
                    }
                    frame 12 {
                      n3046 = Fract/Exp String To Number(string=w4296) -> (number=→"HCF 2":dbl)  [unwired: 3 in, 1 out]
                    }
                    frame 13 {
                      n3047 = Fract/Exp String To Number(string=w4298) -> (number=→"WS1.4 2":dbl)  [unwired: 3 in, 1 out]
                    }
                    frame 14, Default {
                    }
                  }
                }
              }
              frame #2 {
              }
            }
            n3048 = local write "OK Button 16"(FALSE ("OK Button 13")) -> ()
          }
        }
        n3049 = Index Array(array=w3942, index="Select Printer 3") -> (element=w3944:string)
        "Selected Printer" <- w3944
        n3050 = case shown="True" w3939 {
          frame False {
          }
          frame True {
            n3051 = flat-sequence {
              frame #0 {
              }
              frame #1 {
                n3052 = Wait (ms)(milliseconds to wait=u32 100) -> ()  [unwired: 1 out]
              }
              frame #2 {
                n3053 = local write "OK Button 16"(FALSE ("Print 3")) -> ()
              }
            }
          }
        }
        n3054 = case shown="True" "Print" {
          tunnel: w3944 -> [_ w4236]
          frame False {
          }
          frame True {
            (unwired) i16 6 ("width (-)")
            (unwired) "TESTED BY : "
            (unwired) "TESTED DATE :"
            (unwired) "SAMPLE ID : "
            (unwired) "SAMPLE DESIGN : "
            w4194 = "\r"
            w4211 = "\r"
            # "add image"
            n3055 = local read "Sample ID"() -> (w4184:string)
            n3056 = local read "Tested by"() -> (w4187:string)
            n3057 = local read "String 34"() -> (w4174:string)
            n3058 = local read "String 45"() -> (w4154:string)
            n3059 = local read "String 35"() -> (w4169:string)
            n3060 = local read "String 37"() -> (w4167:string)
            n3061 = local read "String 32"() -> (w4189:string)
            n3062 = local read "String 36"() -> (w4164:string)
            n3063 = local read "String 31"() -> (w4188:string)
            n3064 = local read "Test Date"() -> (w4185:string)
            n3065 = local read "String 33"() -> (w4190:string)
            n3066 = local read "String 38"() -> (w4160:string)
            n3067 = local read "String 39"() -> (w4157:string)
            n3068 = local write "Print"(FALSE ("Print FF")) -> ()
            n3069 = local read "S 39"() -> (w4172:string)
            n3070 = local read "S 38"() -> (w4179:string)
            n3071 = local read "Temperature before test 2"() -> (w4210:dbl)
            n3072 = local read "Temperature after test 2"() -> (w4200:dbl)
            n3073 = local read "Humidity before test 2"() -> (w4225:dbl)
            n3074 = local read "Humidity after test 2"() -> (w4209:dbl)
            n3075 = local read "MWSD 2"() -> (w4214:dbl)
            n3076 = local read "WS1.4 2"() -> (w4192:dbl)
            n3077 = Concatenate Strings("2)" ("string"), w4174) -> (w4175:string)
            n3078 = Concatenate Strings("3)" ("string"), w4172) -> (w4173:string)
            n3079 = Concatenate Strings("1)" ("string"), w4179) -> (w4178:string)
            n3080 = Concatenate Strings("4)" ("string"), w4169) -> (w4170:string)
            n3081 = Concatenate Strings("5)" ("string"), w4167) -> (w4166:string)
            n3082 = Concatenate Strings("6)" ("string"), w4164) -> (w4163:string)
            n3083 = Concatenate Strings("7)" ("string"), w4160) -> (w4161:string)
            n3084 = Concatenate Strings("8)" ("string"), w4157) -> (w4158:string)
            n3085 = local read "HCF 2"() -> (w4196:dbl)
            n3086 = local read "AVP 2"() -> (w4213:dbl)
            n3087 = local read "s.NO"() -> (w4155:string)
            n3088 = call <vilib>:"New Report.vi"("report type"=enum16{"Standard Report", "HTML"}."Standard Report") -> ("report out"=w4234:refnum<class "NI_report.lvclass">, "error out"=w4233:errorcluster)  [unwired: 13 in]
            n3089 = local read "TITTLE"() -> (w4186:string)
            n3090 = Concatenate Strings(w4211, w4154, w4155, w4211, w4189, w4184, w4211, w4188, w4185, w4211, w4190, w4187, w4211) -> (w4204:string)
            "test by" <- w4204
            n3091 = Number To Fractional String(number=w4210, width (-)=i16 6, precision (6)=i16 2) -> (F-format string=w4199:string)  [unwired: 1 in]
            n3092 = Number To Fractional String(number=w4209, width (-)=i16 6, precision (6)=i16 2) -> (F-format string=w4212:string)  [unwired: 1 in]
            n3093 = Number To Fractional String(number=w4225, width (-)=i16 6, precision (6)=i16 2) -> (F-format string=w4230:string)  [unwired: 1 in]
            n3094 = Number To Fractional String(number=w4214, width (-)=i16 6, precision (6)=i16 2) -> (F-format string=w4216:string)  [unwired: 1 in]
            n3095 = Number To Fractional String(number=w4200, width (-)=i16 6, precision (6)=i16 2) -> (F-format string=w4201:string)  [unwired: 1 in]
            n3096 = Number To Fractional String(number=w4213, width (-)=i16 6, precision (6)=i16 2) -> (F-format string=w4215:string)  [unwired: 1 in]
            n3097 = Number To Fractional String(number=w4196, width (-)=i16 6, precision (6)=i16 2) -> (F-format string=w4195:string)  [unwired: 1 in]
            n3098 = Number To Fractional String(number=w4192, precision (6)=i16 2) -> (F-format string=w4191:string)  [unwired: 2 in]
            n3099 = call-dynamic "Set Report Header Text.vi"("report in"=w4234, "center header text"=w4186, "error in (no error)"=w4233) -> ("report out"=w4205:refnum<class "NI_report.lvclass">, "error out"=w4206:errorcluster)  [unwired: 11 in]
            n3100 = Concatenate Strings(w4194, w4178, w4230, w4194, w4175, w4199, w4194, w4173, w4212, w4194, w4170, w4201, w4194, w4166, w4216, w4194, w4163, w4215, w4194, w4161, w4195, w4194, w4158, w4191) -> (w4182:string)
            "export 2" <- w4182
            n3101 = call-poly <vilib>:"Append Report Text.vi"("report in"=w4205, "text"=w4204, "error in (no error)"=w4206) -> ("report out"=w4208:refnum<class "NI_report.lvclass">, "error out"=w4207:errorcluster)  [unwired: 9 in, 2 out]
            n3102 = local read "test by"() -> (w4181:string)
            n3103 = local read "TITTLE"() -> (w4183:string)
            n3104 = call-poly <vilib>:"Append Report Text.vi"("report in"=w4208, "error in (no error)"=w4207) -> ("report out"=w4229:refnum<class "NI_report.lvclass">, "error out"=w4227:errorcluster)  [unwired: 10 in, 2 out]
            n3105 = Concatenate Strings(w4183, w4182, w4181) -> (→"output":string)
            n3106 = call-poly <vilib>:"Append Report Text.vi"("report in"=w4229, "text"=w4182, "error in (no error)"=w4227) -> ("report out"=w4228:refnum<class "NI_report.lvclass">, "error out"=w4226:errorcluster)  [unwired: 9 in, 2 out]
            n3107 = call-dynamic "Print Report.vi"("report in"=w4228, "printer name (default)"=w4236, "error in (no error)"=w4226) -> ("report out"=w4238:refnum<class "NI_report.lvclass">, "error out"=w4239:errorcluster)  [unwired: 11 in]
            n3108 = call-dynamic "Dispose Report.vi"("report in"=w4238, "error in (no error)"=w4239) -> ()  [unwired: 13 in, 1 out]
          }
        }
        n3109 = case shown="True" "Print 2" {
          frame False {
          }
          frame True {
            n3110 = flat-sequence {
              frame #0 {
                n3111 = local read "s.NO"() -> (→"s.NO 2":string)
                n3112 = Wait (ms)(milliseconds to wait=u32 20) -> ()  [unwired: 1 out]
                n3113 = local read "Sample ID  3"() -> (→"Sample ID  6":string)
                n3114 = local read "Sample ID  4"() -> (→"Sample ID  7":string)
                n3115 = local read "Sample ID"() -> (→"Sample ID  2":string)
                n3116 = local read "Tested by"() -> (→"Tested by 2":string)
                n3117 = local read "Test Date"() -> (→"Test Date 2":string)
                n3118 = local read "Humidity after test 3"() -> (→"Humidity after test 4":dbl)
                n3119 = local read "Ref A Test Date :"() -> (→"TITTLE 4":string)
                n3120 = local read "Temperature before test 3"() -> (w4061:dbl)
                n3121 = local read "Temperature before test 3"() -> (→"Temperature after test 5":dbl)
                n3122 = local read "Temperature after test 3"() -> (→"Temperature after test 4":dbl)
                n3123 = local read "Humidity before test 3"() -> (→"Humidity before test 4":dbl)
                n3124 = local write "Temperature before test 3"(w4061) -> ()
                n3125 = local read "image data"() -> (w4052:T13)
                n3126 = String To Path(string="C:\\LAB-IQ\\im\\Temp_resized.jpg") -> (path=w4053:path)
                "path 2" <- w4053
                n3127 = call <vilib>:"Write JPEG File.vi"("image data"=w4052, "path to JPEG file"=w4053) -> ()  [unwired: 8 in, 2 out]
                "Ref A Test Date :" <- "Ref A Test Date :"
                "Ref B Test Date :" <- "Ref B Test Date :"
                "Ref B Scar Value :" <- "Ref B Scar Value :"
                "Ref A Scar Value :" <- "Ref A Scar Value :"
              }
              frame #1 {
                (unwired) HTML_Report_Image_Alignment."MIDDLE" ("alignment (default)")
                w4089 = u16 0 items=["portrait", "landscape"] ("orientation (portrait)")
                (unwired) HTML_Report_Image_Alignment."ABSMIDDLE" ("alignment (default)")
                (unwired) "TESTED BY : "
                (unwired) "TESTED DATE :"
                (unwired) "SAMPLE ID : "
                (unwired) "SAMPLE DESIGN : "
                w4122 = "\r"
                # "add image"
                n3128 = Wait (ms)(milliseconds to wait=u32 20) -> ()  [unwired: 1 out]
                n3129 = local read "Sample ID  2"() -> (w4115:string)
                n3130 = local read "Wear Scar X"() -> (w4087:dbl)
                "Length ( microns ) 2" <- w4087
                n3131 = local read "Wear Scar Y"() -> (w4086:dbl)
                "Wear Scar Y ( microns ) :" <- w4086
                n3132 = local read "Test Date 2"() -> (w4116:string)
                n3133 = local read "Tested by 2"() -> (w4117:string)
                n3134 = local read "String 46"() -> (w4113:string)
                n3135 = local read "String 48"() -> (w4119:string)
                n3136 = local read "String 47"() -> (w4118:string)
                n3137 = local read "String 49"() -> (w4120:string)
                n3138 = local read "String 10"() -> (w4073:string)
                n3139 = local read "s.NO 2"() -> (w4114:string)
                n3140 = Add(x=w4087, y=w4086) -> (x+y=w4085:dbl)
                n3141 = call <vilib>:"New Report.vi"("report type"=enum16{"Standard Report", "HTML"}."HTML") -> ("report out"=w4093:refnum<class "NI_report.lvclass">, "error out"=w4091:errorcluster)  [unwired: 13 in]
                n3142 = Concatenate Strings(w4122, w4113, w4114, w4122, w4119, w4115, w4122, w4118, w4116, w4122, w4120, w4117, w4122) -> (→"test by 2":string)
                n3143 = Concatenate Strings("C:\\LAB-IQ\\Data\\" ("string"), w4073, ".jpg" ("string")) -> ()  [unwired: 1 out]
                n3144 = Divide(x=w4085, y=2.0) -> (x/y=→"Mean Wear ( microns) :":dbl)
                n3145 = call-dynamic "Set Report Orientation.vi"("report in"=w4093, "orientation (portrait)"=w4089, "error in (no error)"=w4091) -> ("report out"=w4092:refnum<class "NI_report.lvclass">, "error out"=w4090:errorcluster)  [unwired: 11 in]
                n3146 = for {
                  N: 5 -> [_]
                  tunnel: w4092 -> [w4143]
                  tunnel: [w4142] -> w4071
                  tunnel: w4090 -> [w4141]
                  tunnel: [w4140] -> w4070
                  n3147 = call-dynamic "Set Report Tab Width.vi"("report in"=w4143, "error in (no error)"=w4141) -> ("report out"=w4142:refnum<class "NI_report.lvclass">, "error out"=w4140:errorcluster)  [unwired: 12 in]
